vi "Write Autoscale Delay.vi"(5 "Autoscale Delay":sgl, 9 "GraphChart in":refnum<class "GraphChart.lvclass">) -> (3 "GraphChart out":refnum<class "GraphChart.lvclass">)   [LabVIEW 2014, in "Raspberry Pi Compatible Compiler for LabVIEW.lvlib" / "GraphChart.lvclass"]
uses:
  GraphChart.lvclass
  GraphChart.lvclass/GraphChart.ctl
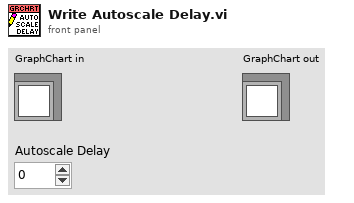
[diagram p1: front panel]
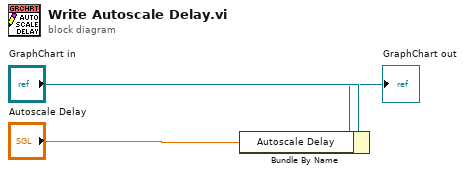
[diagram p0: block diagram]
diagram:
  n1 = Bundle By Name(cluster="GraphChart in", "Autoscale Delay"="Autoscale Delay") -> (→"GraphChart out":refnum<class "GraphChart.lvclass">)
